vi "Get Data Timestamp.vi"(11 "variant in":variant) -> (1 "timestamp":timestamp format="%<%H:%M:%S%6u\n%x>T", 3 "variant out":variant)   [LabVIEW 2017]
uses:
  <vilib>/addons/_NISVFA/_Shared subVIs/Controls/NI Channel Properties.ctl
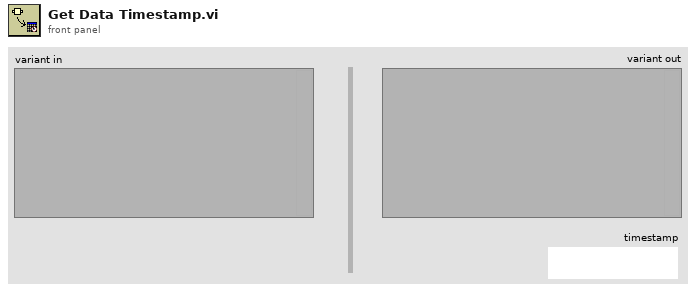
[diagram p1: front panel]
types:
  T1 = typedef "NI Channel Properties.ctl" = u16
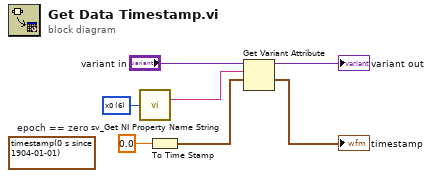
[diagram p0: block diagram]
diagram:
  w4 = T1 6 items=["Channel name", "Channel description", "Axis label", "Unit string", "Waveform X-axis label", "Waveform X-axis unit string", "x0", "dx", "Number of samples", "X channel", "Filter settled", "dB reference", "Window", "Window parameter", "Window size", "FFT size", "Peak units", "Spectrum type", "Magnitude scale", "Spectral density", "Sensor sensitivity (mV/EU)", "X-axis dimension", "LabVIEW datatype", "Function type", "Function subtype", "X values", "Independent channel", "Column index", "Collection name", "Collection ID", "X Columns", "Phase unwrapped"] ("property")
  (unwired) timestamp(0 s since 1904-01-01)  # epoch == zero
  n1 = call <vilib>:"sv_Get NI Property Name String.vi"("property"=w4) -> ("TDMS property name"=w3:string)  [unwired: 13 in, 1 out]
  n2 = To Time Stamp(1:0.0 ("number")) -> (0:w1:timestamp)
  n3 = Get Variant Attribute(Variant="variant in", name=w3, default value (empty Variant)=w1) -> (duplicate Variant=→"variant out":variant, value=→"timestamp":timestamp)  [unwired: 1 in, 2 out]
